vi "state machine.vi"() -> ()   [LabVIEW 2012]
panel:
  out "Enum":enum16{"00", "01", "10", "11"}(ring)
  in  "Boolean":bool
  in  "stop":bool
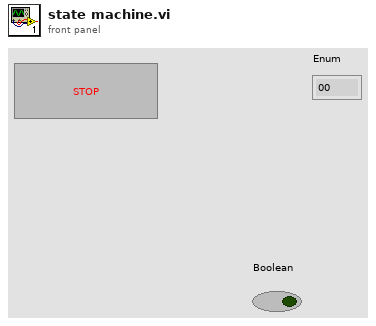
[diagram p1: front panel]
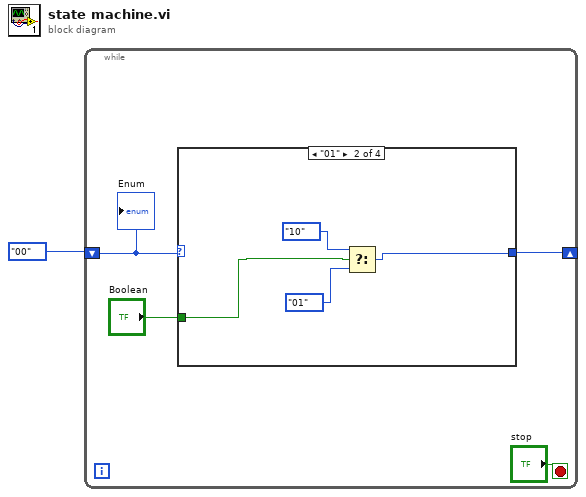
[diagram p0: block diagram]
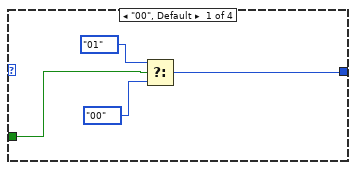
[diagram p2: hidden frame]
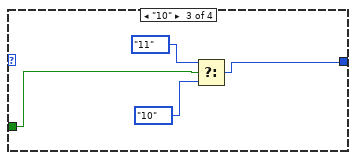
[diagram p3: hidden frame]
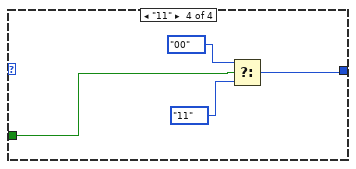
[diagram p4: hidden frame]
diagram:
  n1 = while {
    shift-right: [w3] -> _
    shift-left: enum16{"00", "01", "10", "11"}."00" ("Enum") -> [w2]
    stop <- "stop" stop-if-true
    n2 = case shown="\"01\"" w2 {
      tunnel: "Boolean" -> [w8 w11 w14 w18]
      tunnel: [w9 w10 w15 w19] -> w3
      frame "00", Default {
        n3 = Select(t=enum16{"00", "01", "10", "11"}."01" ("Enum"), s=w8, f=enum16{"00", "01", "10", "11"}."00" ("Enum")) -> (s? t:f=w9:enum16{"00", "01", "10", "11"})
      }
      frame "01" {
        n4 = Select(t=enum16{"00", "01", "10", "11"}."10" ("Enum"), s=w11, f=enum16{"00", "01", "10", "11"}."01" ("Enum")) -> (s? t:f=w10:enum16{"00", "01", "10", "11"})
      }
      frame "10" {
        n5 = Select(t=enum16{"00", "01", "10", "11"}."11" ("Enum"), s=w14, f=enum16{"00", "01", "10", "11"}."10" ("Enum")) -> (s? t:f=w15:enum16{"00", "01", "10", "11"})
      }
      frame "11" {
        n6 = Select(t=enum16{"00", "01", "10", "11"}."00" ("Enum"), s=w18, f=enum16{"00", "01", "10", "11"}."11" ("Enum")) -> (s? t:f=w19:enum16{"00", "01", "10", "11"})
      }
    }
    "Enum" <- w2
  }
